vi "State_Machine.vi"(8 "error in (no error)":errorcluster caption="entrée d'erreur (pas d'erreur)", 11 "Delay en entrée":refnum<class "P2201_Scan_SN.lvclass">) -> (0 "error out":errorcluster caption="sortie d'erreur", 2 "Json_String":string, 3 "Delay en sortie":refnum<class "P2201_Scan_SN.lvclass">)   [LabVIEW 2020, in "Library Test.lvlib" / "P2201_Scan_SN.lvclass"]
uses:
  P2201_Scan_SN.lvclass
  C:/Users/ngarcin/OneDrive - Altyor/Standard TB/Suite TB45/Class/Test/Test (Default)/Test (Default).lvclass
  Popup/Class Popup Operator_Input Batch_AIS/Class Popup Operator_Input_PCRE.lvclass
  Popup/Class Popup (Main)/Class Popup (Main).lvclass
  Commun VI/TypeDef/Variable Printable.ctl
  JSON API/JSON Value/Set from JSON string.vi
  JSON API/JSON Value/JSON Value.lvclass
  JSON API/Variant JSON/Variant JSON.lvlib
  JSON API/Get Polymorphic/JSON GetSet.lvlib
  Commun VI/Library Commun.lvlib
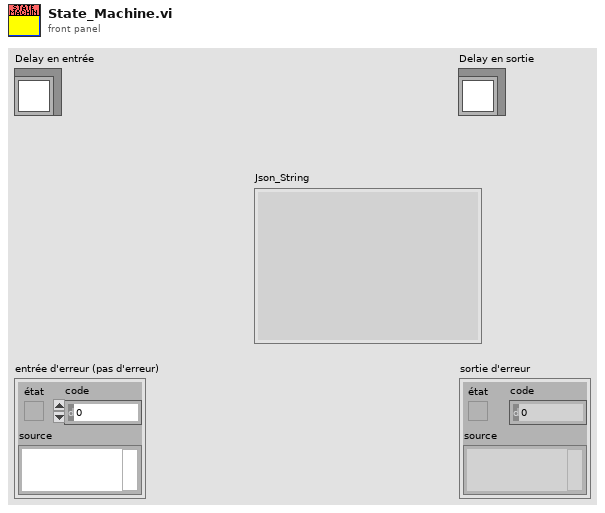
[diagram p1: front panel]
types:
  T1 = typedef "Variable Printable.ctl" = string
  T2 = enum16{"Get Variable", "Get All Variables", "Set Variable", "Delete Variable", "Delete All Variable"}
  T3 = cluster{"Case_ID":string, "SN_Product":string, "Model_Product":string, "Certificate_Number":string}
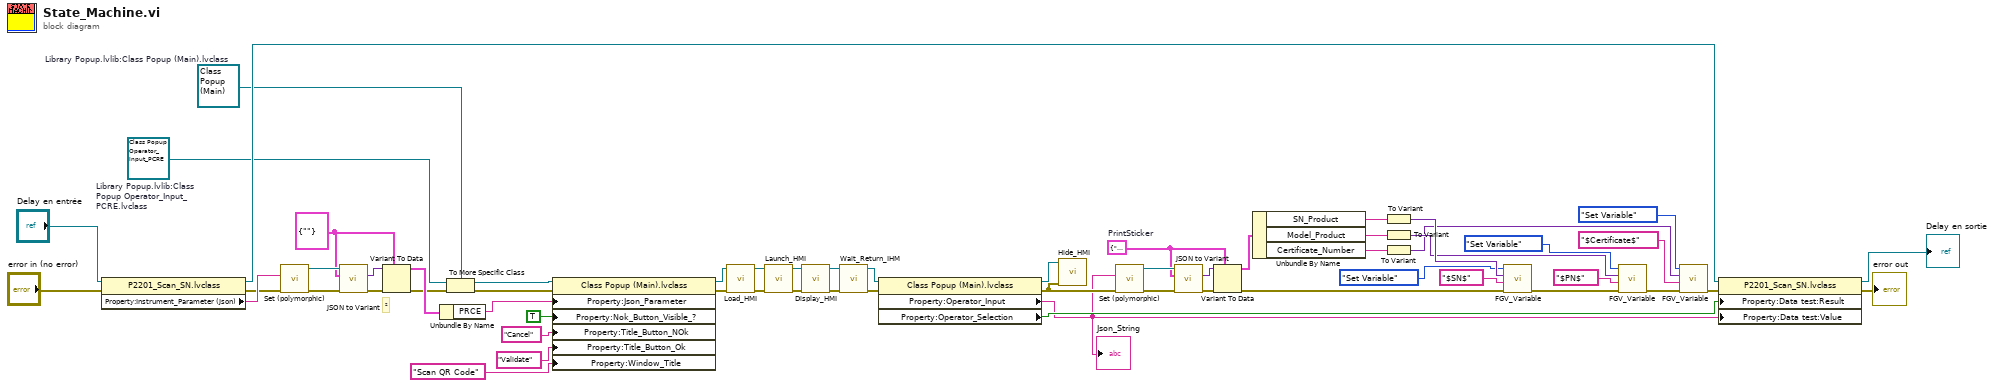
[diagram p0: block diagram]
diagram:
  w16 = T3 {"Case_ID"="", "SN_Product"="", "Model_Product"="", "Certificate_Number"=""}  # PrintSticker
  w31 = refnum<class "Class Popup (Main).lvclass"> refnum  # Library Popup.lvlib:Class Popup (Main).lvclass
  w34 = cluster{"PRCE":string} {"PRCE"=""}
  w30 = refnum<class "Class Popup Operator_Input_PCRE.lvclass"> refnum  # Library Popup.lvlib:Class Popup Operator_Input_PCRE.lvclass
  # "²"
  n1 = property class="P2201_Scan_SN.lvclass"(reference="Delay en entrée", error in="error in (no error)") -> (reference out=w40:refnum<class "P2201_Scan_SN.lvclass">, error out=w56:errorcluster, "Property:Instrument_Parameter (Json)"=w58:string)
  n2 = call-poly "Set (polymorphic).vi"("error in (no error)"=w56, "JSON stream"=w58) -> ("error out"=w36:errorcluster, "JSON Value out"=w38:refnum<class "JSON Value.lvclass">)  [unwired: 7 in, 1 out]
  n3 = call "JSON to Variant.vi"("error in (no error)"=w36, "Variant (Data Type)"=w34, "JSON Value"=w38) -> ("error out"=w37:errorcluster, "Variant out"=w35:variant)  [unwired: 7 in]
  n4 = Variant To Data(error in=w37, type=w34, Variant=w35) -> (data=w33:cluster{"PRCE":string}, error out=w28:errorcluster)
  n5 = Unbundle By Name(w33) -> ("PRCE"=w32:string)
  n6 = To More Specific Class(target class=w31, reference=w30, error in=w28) -> (specific class reference=w29:refnum<class "Class Popup (Main).lvclass">, error out=w27:errorcluster)
  n7 = property class="Class Popup (Main).lvclass"(reference=w29, error in=w27, "Property:Json_Parameter"=w32, "Property:Nok_Button_Visible_?"=TRUE ("Nok_Button_Visible_?"), "Property:Title_Button_NOk"="Cancel" ("Title_Button_NOk"), "Property:Title_Button_Ok"="Validate" ("Title_Button_Ok"), "Property:Window_Title"="Scan QR Code" ("Window_Title")) -> (reference out=w50:refnum<class "Class Popup (Main).lvclass">, error out=w49:errorcluster)
  n8 = call-dynamic "Load_HMI.vi"("error in (no error)"=w49, "Class Popup (Default) en entrée"=w50) -> ("error out"=w55:errorcluster, "Class Popup (Default) en sortie"=w54:refnum<class "Class Popup (Main).lvclass">)  [unwired: 8 in]
  n9 = call-dynamic "Launch_HMI.vi"("error in (no error)"=w55, "Class Popup (Default) en entrée"=w54) -> ("error out"=w53:errorcluster, "Class Popup (Default) en sortie"=w52:refnum<class "Class Popup (Main).lvclass">)  [unwired: 8 in]
  n10 = call-dynamic "Display_HMI.vi"("error in (no error)"=w53, "Class Popup (Default) en entrée"=w52) -> ("error out"=w25:errorcluster, "Class Popup (Default) en sortie"=w51:refnum<class "Class Popup (Main).lvclass">)  [unwired: 8 in]
  n11 = call-dynamic "Wait_Return_IHM.vi"("error in (no error)"=w25, "Class Popup (Default) en entrée"=w51) -> ("error out"=w26:errorcluster, "Class Popup (Default) en sortie"=w45:refnum<class "Class Popup (Main).lvclass">)  [unwired: 8 in]
  n12 = property class="Class Popup (Main).lvclass"(reference=w45, error in=w26) -> (reference out=w44:refnum<class "Class Popup (Main).lvclass">, error out=w17:errorcluster, "Property:Operator_Input"=w12:string, "Property:Operator_Selection"=w39:bool)
  "Json_String" <- w12
  n13 = call-dynamic "Hide_HMI.vi"("error in (no error)"=w17, "Class Popup (Default) en entrée"=w44) -> ()  [unwired: 8 in, 2 out]
  n14 = call-poly "Set (polymorphic).vi"("error in (no error)"=w17, "JSON stream"=w12) -> ("error out"=w19:errorcluster, "JSON Value out"=w21:refnum<class "JSON Value.lvclass">)  [unwired: 7 in, 1 out]
  n15 = call "JSON to Variant.vi"("error in (no error)"=w19, "Variant (Data Type)"=w16, "JSON Value"=w21) -> ("error out"=w20:errorcluster, "Variant out"=w18:variant)  [unwired: 7 in]
  n16 = Variant To Data(error in=w20, type=w16, Variant=w18) -> (data=w15:T3, error out=w14:errorcluster)
  n17 = Unbundle By Name(w15) -> ("SN_Product"=w13:string, "Model_Product"=w3:string, "Certificate_Number"=w2:string)
  n18 = To Variant(anything=w13) -> (Variant=w24:variant)
  n19 = To Variant(anything=w3) -> (Variant=w9:variant)
  n20 = To Variant(anything=w2) -> (Variant=w7:variant)
  n21 = call "FGV_Variable.vi"("error in (no error)"=w14, "Variable"=T1 "$SN$", "Data In"=w24, "Function"=T2."Set Variable") -> ("error out"=w8:errorcluster)  [unwired: 5 in, 2 out]
  n22 = call "FGV_Variable.vi"("error in (no error)"=w8, "Variable"=T1 "$PN$", "Data In"=w9, "Function"=T2."Set Variable") -> ("error out"=w5:errorcluster)  [unwired: 5 in, 2 out]
  n23 = call "FGV_Variable.vi"("error in (no error)"=w5, "Variable"=T1 "$Certificate$", "Data In"=w7, "Function"=T2."Set Variable") -> ("error out"=w4:errorcluster)  [unwired: 5 in, 2 out]
  n24 = property class="P2201_Scan_SN.lvclass"(reference=w40, error in=w4, "Property:Data test:Result"=w39, "Property:Data test:Value"=w12) -> (reference out=→"Delay en sortie":refnum<class "P2201_Scan_SN.lvclass">, error out=→"error out":errorcluster)
